vi "Decorate.vi"(10 "Actor":refnum<class "Actor.lvclass">, 11 "TEMPLATE Actor in":refnum<class "{{Name}}Actor.lvclass">) -> (3 "TEMPLATE Actor out":refnum<class "{{Name}}Actor.lvclass">)   [LabVIEW 2020, in "_Template.lvlib" / "Templates.lvlib" / "{{Name}}Actor.lvlib" / "{{Name}}Actor.lvclass"]
uses:
  {{Name}}Actor.lvclass
  {{Name}}Actor.lvclass/{{Name}}Actor.ctl
  jettl/jettl/Actor/Actor.lvclass
panel:
  # "This front panel should not be manipulated."
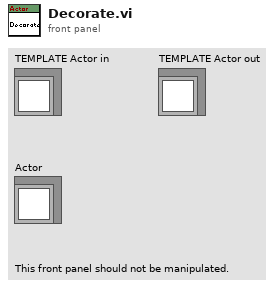
[diagram p1: front panel]
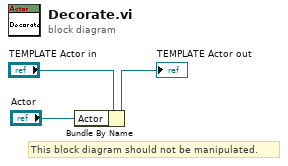
[diagram p0: block diagram]
diagram:
  # "This block diagram should not be manipulated."
  n1 = Bundle By Name(cluster="TEMPLATE Actor in", "Actor"="Actor") -> (→"TEMPLATE Actor out":refnum<class "{{Name}}Actor.lvclass">)
